vi "Build_Erd_Header_Name_And_Number.vi"(5 "ERD Name Array In":string[](array[string]), 7 "ERD Number Array In":string[](array[string])) -> (6 "Header_To_Write":string[][](array[string]))   [LabVIEW 2023]
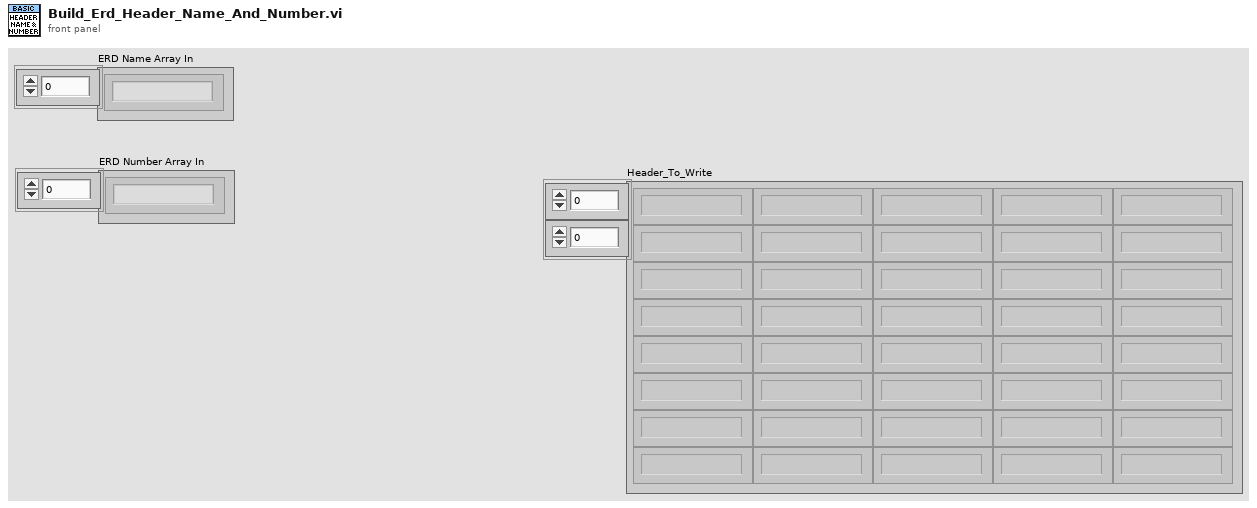
[diagram p1: front panel]
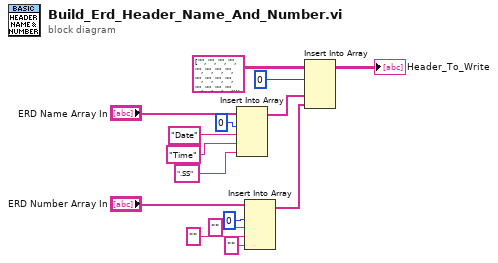
[diagram p0: block diagram]
diagram:
  n1 = Insert Into Array(array="ERD Name Array In", index=0, new element #1="Date", new element #2="Time", new element #3=".SS" ("new element/subarray")) -> (w3:string[])
  n2 = Insert Into Array(array="ERD Number Array In", index=0, new element #1="" ("new element/subarray"), new element #2="" ("new element/subarray"), new element #3="" ("new element/subarray")) -> (w2:string[])
  n3 = Insert Into Array(array=string[][] [["", "", "", "", "", "", "", "", "", "", "", "", "", "", "", "", "", "", "", "", "", "", "", "", "", "", "", "", "", "", "", "", "", "", "", "", "", "", "", "", "", "", "", "", "", "", "", "", "", "", "", "", "", "", "", "", "", "", "", "", "", "", "", "", "", "", "", "", "", "", "", "", "", "", "", "", "", "", "", "", "", "", "", "", "", "", ""]] ("Array Ini"), index (row)=0, new element #1=w3, new element #2=w2) -> (→"Header_To_Write":string[][])  [unwired: 1 in]
